vi "GUI.Disable.vi"(7 "VI reference (current VI)":refnum<vi>, 8 "error in (no error)":errorcluster, 11 "Array":refnum<vi>[](array[refnum])) -> (0 "error out":errorcluster)   [LabVIEW 2015]
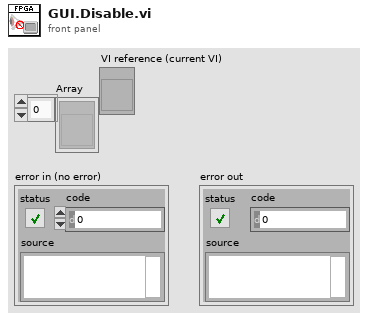
[diagram p1: front panel]
types:
  T1 = enum8{"Enabled", "Disabled", "Disabled and Grayed Out"}
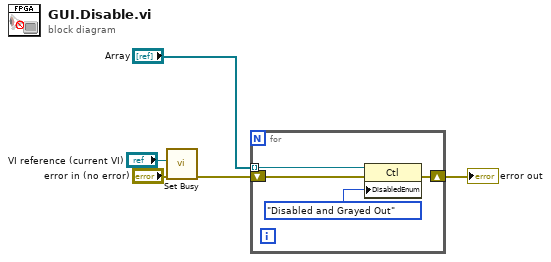
[diagram p0: block diagram]
diagram:
  n1 = call <vilib>:"Set Busy.vi"("error in (no error)"="error in (no error)", "VI reference (current VI)"="VI reference (current VI)") -> ("error out"=w5:errorcluster)  [unwired: 8 in, 1 out]
  n2 = for {
    tunnel: "Array" -> [w9] mode=indexing
    shift-right: [w6] -> w2
    shift-left: w5 -> [w7]
    n3 = property class="Ctl"(reference=w9, error in=w7, "DisabledEnum"=T1."Disabled and Grayed Out" ("Disabled")) -> (error out=w6:errorcluster)  [unwired: 1 out]
  }
  "error out" <- w2
